vi "二维动态避障简单测试0607(远程版)).vi"() -> ()   [LabVIEW 2018]
doc: "Demonstrates the use of the Network Streams functions to send LED status to the myRIO target."
uses:
  <vilib>/addons/zeromq/socket_type.ctl
  <vilib>/ErrorRing/Error Ring.xnode
  <vilib>/vision/NI_Vision_Development_Module.lvlib
  <vilib>/addons/zeromq/zmq_socket.lvclass
  <vilib>/addons/zeromq/zmq_context.lvclass
  <vilib>/addons/zeromq/zeromq.lvlib
panel:
  in  "start_x手动输入":ext=863.0
  in  "start_y手动输入":ext=497.0
  out "start_point_x 2(opencv判断)":ext
  out "start_point_y 2(opencv判断)":ext
  out "c2":ext
  out "c1":ext
  out "next_relative_desired_point_y":ext
  out "next_relative_desired_point_x":ext
  in  "簇 14":cluster{"c1":ext, "c2":ext}={"c1"=100000.0, "c2"=100000.0}
  out "relative_real_y_color 2":dbl=2.0
  out "relative_real_x_color 2":dbl=2.0
  in  "簇 13":T1={"relative_real_x_color"=100000.0, "relative_real_y_color"=1.0, "t"=1.0}
  out "u(t)_y":ext
  out "u(t)_x":ext
  out "relative_real_y_color":ext
  out "relative_real_x_color":ext
  in  "中心轨迹":bool
  in  "打开彩色点轨迹":bool
  out "relative_real_y_color":ext
  out "relative_real_x_color":ext
  out "彩色轨迹":T2(plugin-control)
  out "end_point_y":ext
  out "end_point_x":ext
  out "end_point_y绝对坐标(opencv拟合)":ext
  out "end_point_x绝对坐标(opencv拟合)":ext
  out "c":ext
  in  "簇 10":T3={"c"=100000.0, "cx"=100000.0, "cy"=100000.0, "start_point_x"=100000.0, "start_point_y"=100000.0}
  out "输出簇":T4
  in  "簇 9":T4={"a"=[], "b"=1.0, "a2"=[], "left1"=1.0, "top1"=1.0, "left2"=1.0, "top2"=1.0, "delta1"=1.0, "delta2"=1.0}
  in  "delta2":dbl=80.0
  out "bottom2":dbl
  out "right2":dbl
  out "top2":dbl
  out "left2":dbl
  in  "delta1":dbl=130.0
  out "bottom1":dbl
  out "right1":dbl
  out "top1":dbl
  out "left1":dbl
  out "delta_pr":dbl
  out "delta_dr":dbl
  in  "k2":dbl=-0.3
  in  "K1":dbl=0.3
  in  "Operation":T5(ring)=enum."Erode"
  out "old_real_relative_point_y":dbl
  out "old_real_relative_point_x":dbl
  out "real_relative_start_point_y":dbl
  out "real_relative_start_point_x":dbl
  out "Bounding Box.Y Top 2":i32
  out "Bounding Box.X Left 2":i32
  out "Ki part":dbl
  out "Kd part":dbl
  out "Kp part":dbl
  out "Ki part":dbl
  out "Kd part":dbl
  out "Kp part":dbl
  in  "Ki":dbl=0.004
  in  "Kd":dbl=5e-05
  in  "Kp":dbl=0.023
  in  "Ki":dbl=0.0035
  in  "Kd":dbl=5e-05
  in  "Kp":dbl=0.023
  out "添加的数组":dbl[](array[numeric])
  out "desired_relative_point_y":dbl=820.0
  out "desired_relative_point_x":dbl=730.0
  out "MLP_pr":dbl=20.0
  out "MLP_dr":dbl=8.0
  out "error_relative_point_y":dbl
  out "error_relative_point_x":dbl
  out "real_relative_end_point_y":dbl
  out "real_relative_end_point_x":dbl
  out "magnet_input_pr":dbl
  out "magnet_input_dr":dbl
  in  "打开仅尖端轨迹":bool
  out "仅尖端轨迹":T2(plugin-control)
  out "Bounding Box.Y Top":i32
  out "Bounding Box.X Left":i32
  out "curve_min_y":dbl
  out "curve_min_x":dbl
  out "curve_max_y":dbl
  out "curve_max_x":dbl
  out "relative_end_point_y":dbl
  out "relative_end_point_x":dbl
  out "delta_y":dbl
  out "delta_x":dbl
  out "pr":dbl=-28.0
  out "tan(v)":dbl
  out "delta_velocity":dbl format="%#_10g"
  out "delta_time":dbl
  out "now time":timestamp[](array[timestamp])
  out "prev time":timestamp[](array[timestamp])
  out "delta_distance":dbl
  out "prev_end_point_y":dbl
  out "prev_end_point_x":dbl
  out "now_end_point_y(曲线拟合)":dbl
  out "now_end_point_x(曲线拟合)":dbl
  out "prev_end_point_y":dbl[](array[numeric])
  out "prev_end_point_x":dbl[](array[numeric])
  out "dr":dbl=120.0
  in  "Ar":sgl=11.0
  out "all parameters":dbl[][](array[numeric])
  out "direction angle":sgl[](array[numeric])
  out "dr":sgl
  out "strength":dbl[](array[numeric])
  out "场强":dbl
  out "end_point_y":T6
  out "end_point_x":dbl[](array[numeric])
  out "start_point_y":dbl[](array[numeric])
  out "start_point_x":dbl[](array[numeric])
  out "T":i32[](array[numeric])
  out "c":dbl[](array[numeric])
  out "b":dbl[](array[numeric])
  out "a\na":dbl[](array[numeric])
  out "c":dbl
  out "b":dbl
  out "a":dbl
  out "Angles (deg)":sgl[](array[numeric]) format="%.2f"
  in  "wr":sgl
  in  "打开轨迹":bool
  out "中心轨迹和尖端轨迹":T2(plugin-control)
  out "end_y绝对坐标(曲线拟合)":dbl
  out "end_x绝对坐标(曲线拟合)":dbl
  out "start_y绝对坐标(曲线拟合)":dbl
  out "start_x绝对坐标(曲线拟合)":dbl
  out "Image Pixels (U8)":u8[][](array[numeric])
  in  "Poly":dbl
  out "中心轨迹":T2(plugin-control)
  in  "保存按钮":bool
  out "Object Center":cluster{"X":sgl, "Y":sgl}
  out "黑白图":T2(plugin-control)
  in  "Number of Erosion":i32=5
  in  "Settings":T7={"Objects"=1, "Threshold"=128, "Reject Border"=FALSE, "Fill Holes"=FALSE, "Min Object Size"=TRUE, "Min Size"=1200, "Max Object Size"=FALSE, "Max Size"=100, "Show Search Area"=TRUE, "Show Center"=TRUE, "Show Bounding Box"=TRUE} {"Objects" items=["Bright Objects", "Dark Objects"]; "Threshold" min=1 max=999999999 step=1; "Max Size" min=1 max=999999999 step=1; "Min Size" min=1 max=999999999 step=1}
  out "Objects":T8(array[cluster]) {"Aspect Ratio" format="%.2f"; "Orientation" format="%.2f"; "Area" format="%.2f"; "Object Center"."Y" format="%.2f"; "Object Center"."X" format="%.2f"}
  in  "Search Rect (entire image)":T9={"Left"=350, "Top"=20, "Right"=1040, "Bottom"=1030, "Rotation"=0.0} {"Rotation" format="%.2f"; "Left" scale=0.0..1024.0; "Right" scale=0.0..1024.0}
  in  "Range":cluster{"Lower value":sgl, "Upper value":sgl}={"Lower value"=177.0, "Upper value"=255.0} {"Upper value" format="%.2f"; "Lower value" format="%.2f"}
  out "原图":T2(plugin-control)
  in  "停止":bool
  out "T":i32
  out "T":i32
  in  "磁场变换":bool=TRUE
  in  "Pause":bool
  out "Array":ext[](array[numeric])
  in  "Parameter Settings":T10(tab)=enum."Rotating Field" caption="Field Types"
  in  "Ag":dbl
  in  "dg":dbl
  in  "pg":dbl
  in  "fg":dbl
  in  "AoOF":dbl
  in  "fo":sgl
  in  "do":sgl
  in  "oo":sgl
  in  "po":sgl
  in  "cc":sgl
  in  "pc":sgl
  in  "wc":sgl
  in  "dc":sgl
  in  "Ac":dbl
  in  "Dis phase step":dbl
  in  "Dis phase frequency (Hz)":dbl
  in  "Dis tumbling frequency (Hz)":dbl
  in  "Dis strength(mT)":dbl
  in  "Swa strength (mT)":dbl
  in  "Swa frequency (Hz)":dbl
  in  "Swa pitch angle (deg)":dbl
  in  "Swa direction angle (deg)":dbl
  in  "Swa ratio":dbl=1.0
  in  "Pitch Angle (rotating around Constant, deg)":dbl
  in  "Ratio (A/C)":sgl
  in  "Direction Angle (deg)":sgl
  in  "Pitch Angle (rotating around Origin, deg)":sgl
  in  "Frequency (Hz)":sgl
  in  "Strength (mT)":dbl
  in  "Ar 2":dbl caption="Ar"
  in  "ratio":sgl
  in  "pr  2":sgl
  in  "dr  2":sgl
  in  "wr  2":sgl
  in  "p_x":sgl
  out "Numeric 5":i32
  in  "Stop":bool
  out "error out":errorcluster
  in  "Target IP Address":string="172.22.11.2"
  # "Overview: Magnetic field calculation, and send parameters to myRIO\nInstructions:\n1. Verify the value of Target IP Address. Set Visa resource name.\n2. Ensure RT Main.vi is already running. \n3. Run this VI. Set parameters of magnetic field."
  # "Strength (mT)"
  # "Frequency (Hz)"
  # "Pitch Angle (deg)"
  # "Direction Angle (deg)"
  # "Strength (mT)"
  # "Pitch Angle (deg)"
  # "Direction Angle (deg)"
  # "Frequency (Hz)"
  # "Strength (mT)"
  # "Oscilation Frequency (Hz)"
  # "Oscilation Angle (deg)"
  # "Pitch Angle (deg)"
  # "Direction Angle (deg)"
  # "Strength (mT)"
  # "Frequency (Hz)"
  # "Pitch Angle (deg)"
  # "Direction Angle (deg)"
  # "Conical Angle (deg)"
  # "Strength (mT)"
  # "Tumbling Frequency (Hz)"
  # "Phase Frequency (Hz)"
  # "Phase Step"
  # "Strength (mT)"
  # "Frequency (Hz)"
  # "Pitch Angle (deg)"
  # "Direction Angle (deg)"
  # "Ratio"
  # "Strength (mT)"
  # "Frequency (Hz)"
  # "Ratio (A/C)"
  # "Direction Angle (deg)"
  # "Pitch Angle (rotating around Origin, deg)"
  # "Pitch Angle (rotating around Constant, deg)"
  # "Strength (mT)"
  # "Frequency (Hz)"
  # "Pitch Angle Y (deg)"
  # "Pitch Angle X (deg)"
  # "Direction Angle (deg)"
  # "ratio (l/s)"
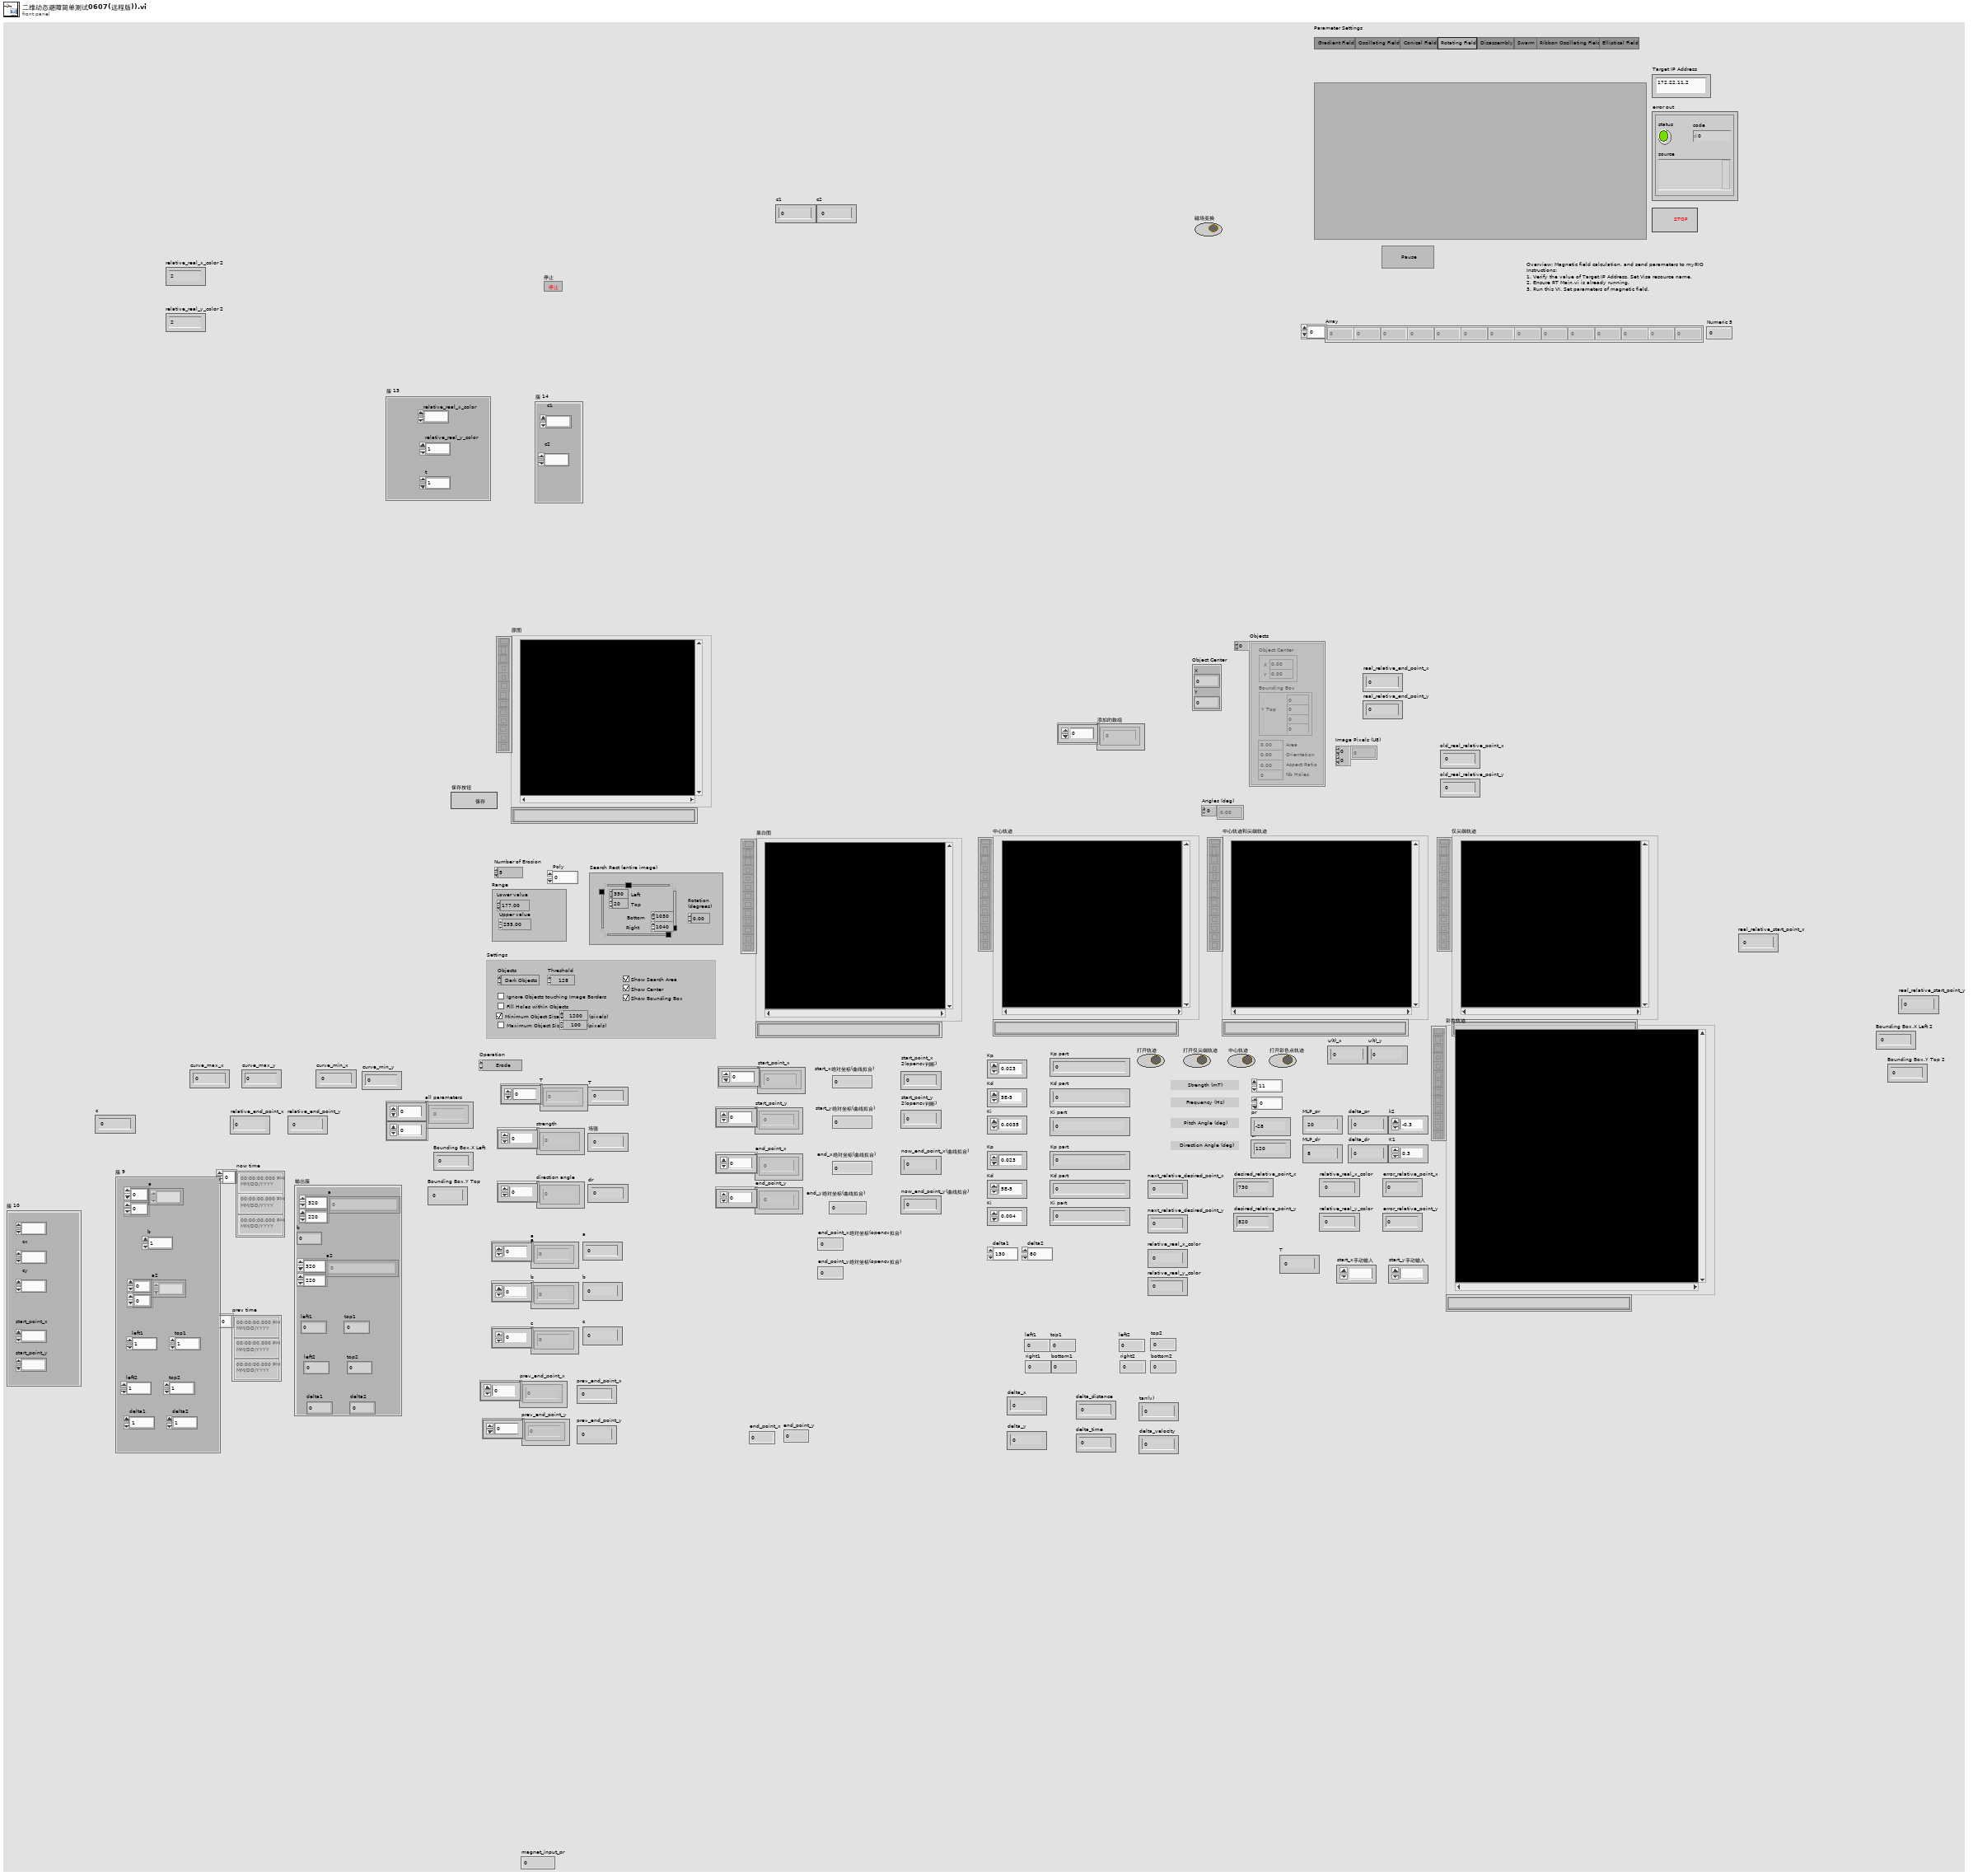
[diagram p1: front panel]
types:
  T1 = cluster{"relative_real_x_color":ext, "relative_real_y_color":dbl, "t":dbl}
  T2 = typedef "IMAQ Image.ctl" = refnum<image>
  T3 = cluster{"c":ext, "cx":ext, "cy":ext, "start_point_x":ext, "start_point_y":ext}
  T4 = cluster{"a":ext[][], "b":dbl, "a2":ext[][], "left1":dbl, "top1":dbl, "left2":dbl, "top2":dbl, "delta1":dbl, "delta2":dbl}
  T5 = enum32{"AutoM", "Close", "Dilate", "Erode", "Gradient", "Gradient in", "Gradient out", "HitMiss", "Open", "PClose", "POpen", "Thick", "Thin"}
  T6 = typedef "控件 3.ctl" = dbl[]
  T7 = cluster{"Objects":u16, "Threshold":i32, "Reject Border":bool, "Fill Holes":bool, "Min Object Size":bool, "Min Size":i32, "Max Object Size":bool, "Max Size":i32, "Show Search Area":bool, "Show Center":bool, "Show Bounding Box":bool}
  T8 = cluster{"Object Center":cluster{"X":sgl, "Y":sgl}, "Bounding Box":cluster{"X Left":i32, "Y Top":i32, "X Right":i32, "Y Bottom":i32}, "Area":sgl, "Orientation":sgl, "Aspect Ratio":sgl, "Nb Holes":i32}[]
  T9 = typedef "IMAQ Rectangle" = cluster{"Left":i32, "Top":i32, "Right":i32, "Bottom":i32, "Rotation":dbl}
  T10 = enum32{"Gradient Field ", "Oscillating Field", "Conical Field", "Rotating Field", "Disassembly", "Swarm", "Ribbon Oscillating Field", "Elliptical Field"}
  T11 = typedef "zeromq.lvlib/socket_type.ctl" = enum8{"ZMQ_PAIR", "ZMQ_PUB", "ZMQ_SUB", "ZMQ_REQ", "ZMQ_REP", "ZMQ_DEALER", "ZMQ_ROUTER", "ZMQ_PULL", "ZMQ_PUSH", "ZMQ_XPUB", "ZMQ_XSUB", "ZMQ_STREAM", "ZMQ_SERVER", "ZMQ_CLIENT", "ZMQ_RADIO", "ZMQ_DISH", "ZMQ_GATHER", "ZMQ_SCATTER", "ZMQ_DGRAM"}
  T12 = typedef "Image Type" = u32
  T13 = cluster{"Object Center":cluster{"X":sgl, "Y":sgl}, "Bounding Box":cluster{"X Left":i32, "Y Top":i32, "X Right":i32, "Y Bottom":i32}, "Area":sgl, "Orientation":sgl, "Aspect Ratio":sgl, "Nb Holes":i32}
  T14 = cluster{"X Left":i32, "Y Top":i32, "X Right":i32, "Y Bottom":i32, "Rotation":dbl}
  T15 = typedef "ROI Descriptor" = cluster{"Global Rectangle":i32[], "Contours":cluster{"ID":enum32{"External", "Internal"}, "Type":u32, "Coordinates":i32[]}[]}
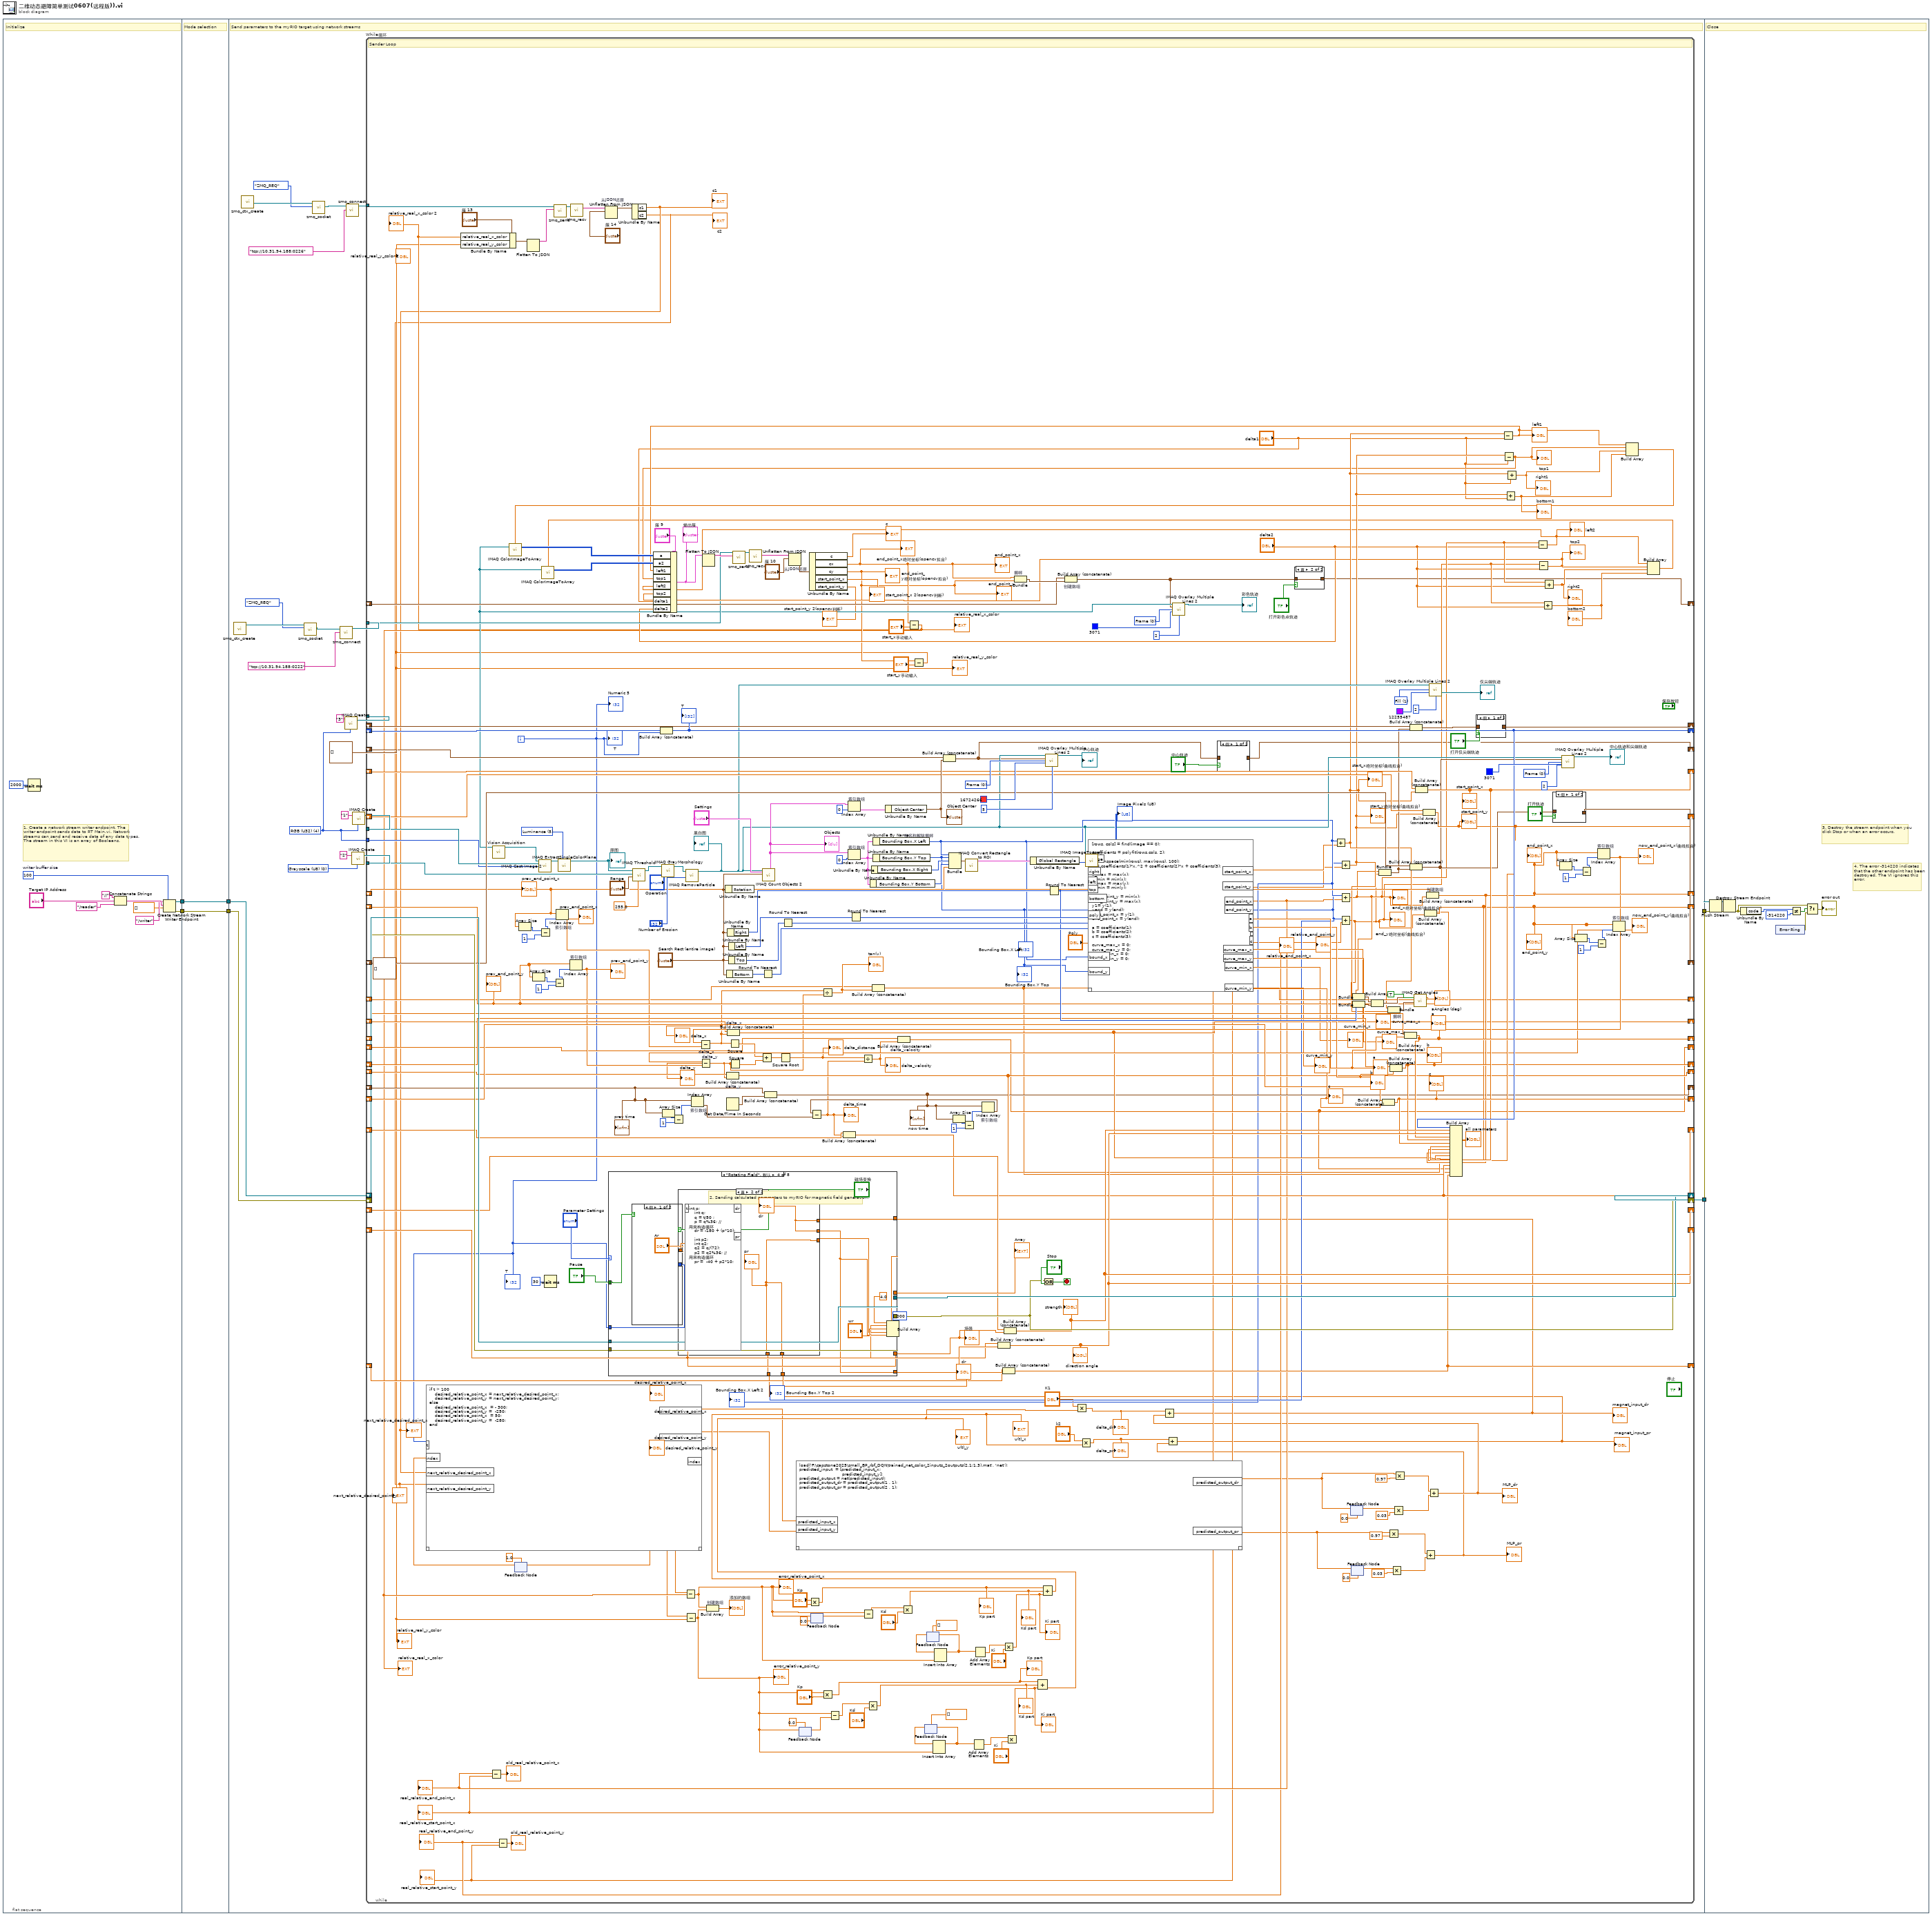
[diagram p0: block diagram]
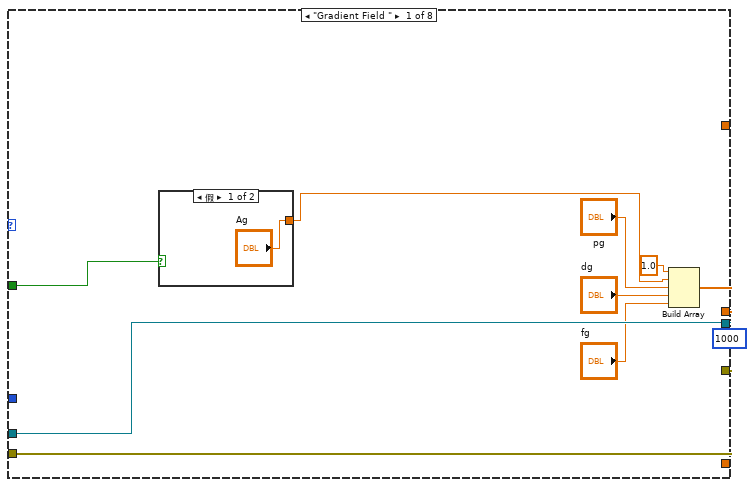
[diagram p6: hidden frame]
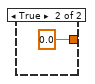
[diagram p7: hidden frame]
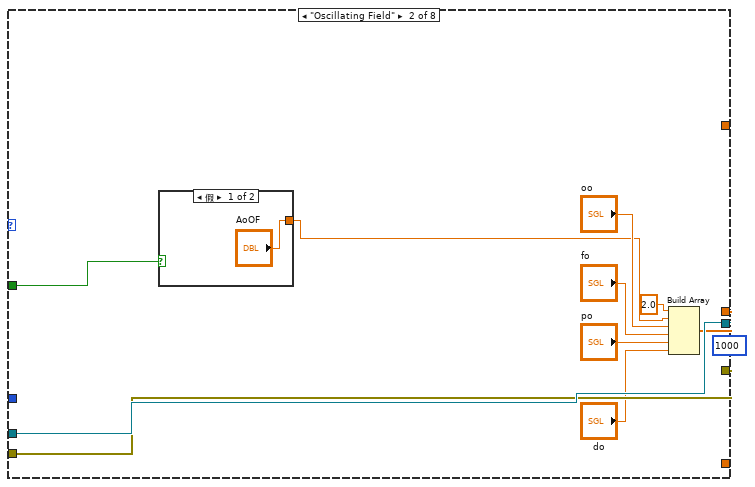
[diagram p8: hidden frame]
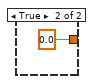
[diagram p9: hidden frame]
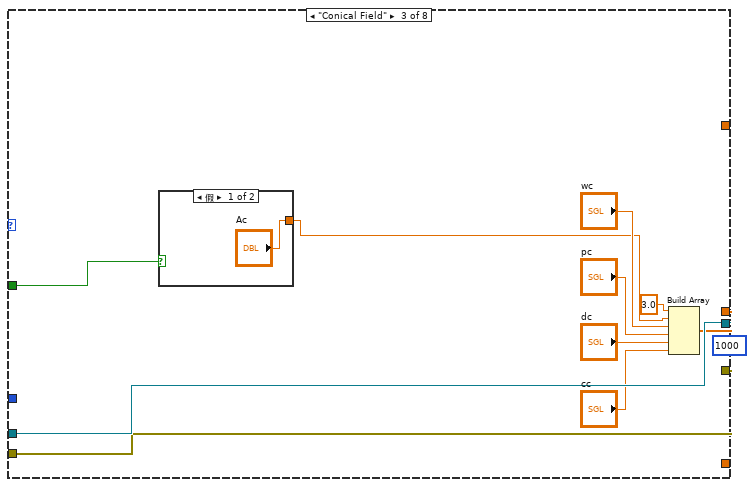
[diagram p10: hidden frame]
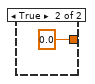
[diagram p11: hidden frame]
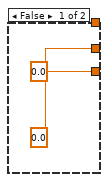
[diagram p12: hidden frame]
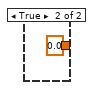
[diagram p13: hidden frame]
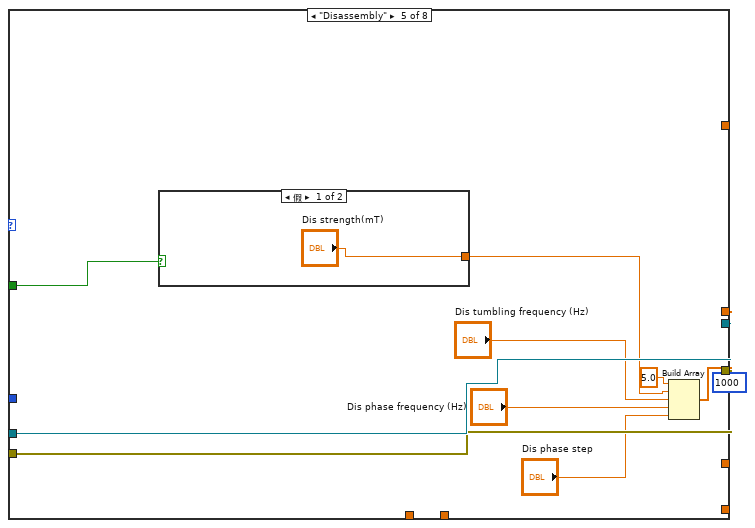
[diagram p14: hidden frame]
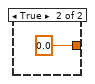
[diagram p15: hidden frame]
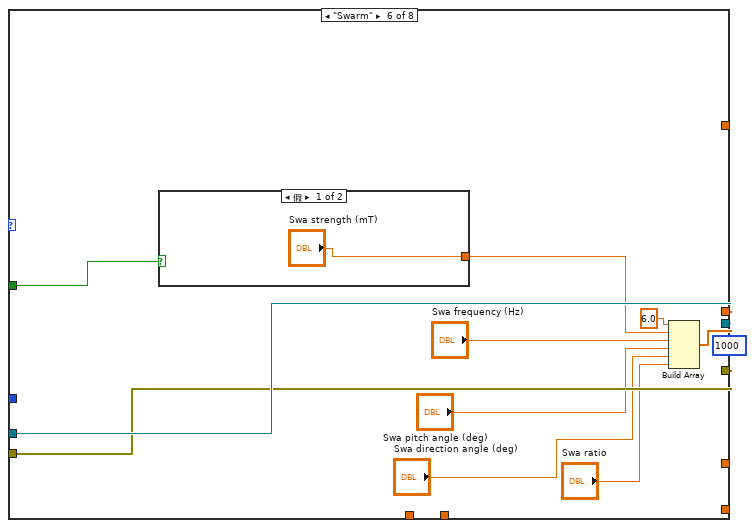
[diagram p16: hidden frame]
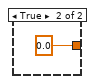
[diagram p17: hidden frame]
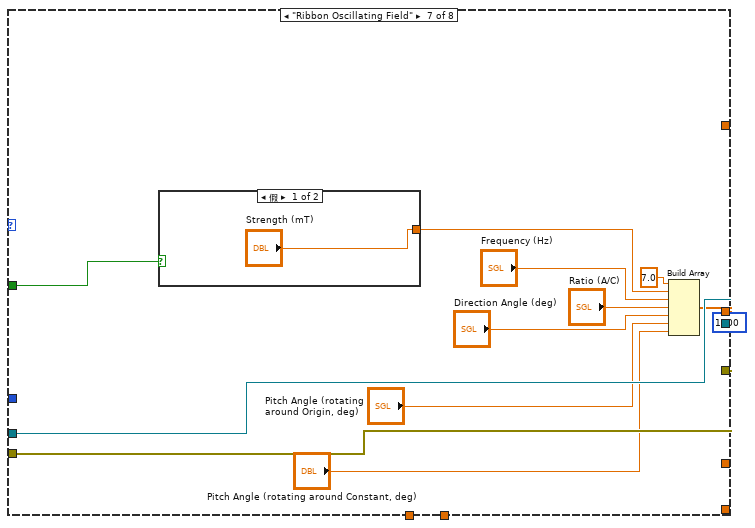
[diagram p18: hidden frame]
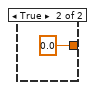
[diagram p19: hidden frame]
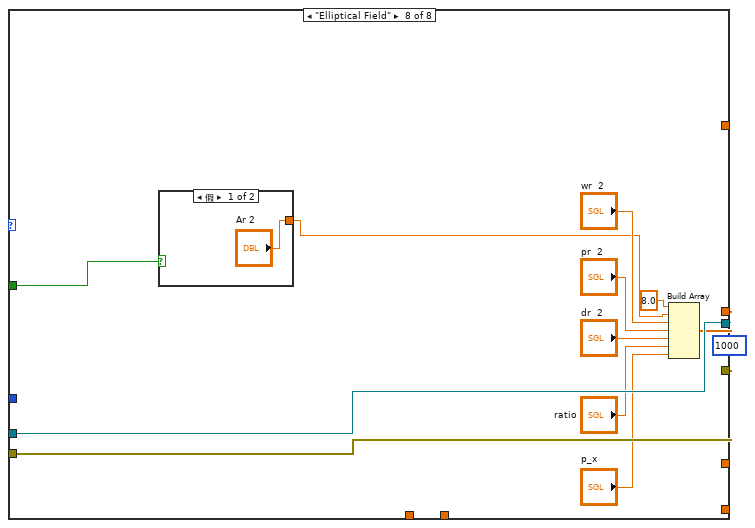
[diagram p20: hidden frame]
diagram:
  n1 = flat-sequence {
    tunnel: [w11] -> w2
    tunnel: [w10] -> w1
    tunnel: [w18] -> w4
    tunnel: [w17] -> w3
    tunnel: w1 -> [w17]
    tunnel: w2 -> [w18]
    tunnel: [w40] -> w6
    tunnel: w4 -> [w42]
    tunnel: [w39] -> w5
    tunnel: w3 -> [w41]
    tunnel: w6 -> [w464]
    tunnel: w5 -> [w461]
    frame #0 {
      w9 = 100  # writer buffer size
      # "1. Create a network stream writer endpoint. The writer endpoint sends data to RT Main.vi. Network streams can send and receive data of any data types. The stream in this VI is an array of Booleans."
      # "Initialize"
      n2 = Wait (ms)(milliseconds to wait=2000) -> ()  [unwired: 1 out]
      n3 = Concatenate Strings("//", "Target IP Address", "/reader") -> (w16:string)
      n4 = Create Network Stream Writer Endpoint(7:w9, 9:dbl[] [], 10:w16, 11:"/writer" ("reader name")) -> (0:w10:errorcluster, 3:w11:refnum<k21>)  [unwired: 3 in]
    }
    frame #1 {
      # "Mode selection"
    }
    frame #2 {
      w36 = T12 0 items=["Grayscale (U8)", "Grayscale (I16)", "Grayscale (SGL)", "Complex (CSG)", "RGB (U32)", "HSL (U32)", "RGB (U64)", "Grayscale (U16)"] ("Image Type")
      w29 = T12 4 items=["Grayscale (U8)", "Grayscale (I16)", "Grayscale (SGL)", "Complex (CSG)", "RGB (U32)", "HSL (U32)", "RGB (U64)", "Grayscale (U16)"] ("Image Type")
      # "Send parameters to the myRIO target using network streams"
      n5 = call <vilib>:"zmq_ctx_create.vi"() -> ("context out"=w27:refnum<class "zmq_context.lvclass">)  [unwired: 4 in, 1 out]
      n6 = call <vilib>:"zmq_ctx_create.vi"() -> ("context out"=w22:refnum<class "zmq_context.lvclass">)  [unwired: 4 in, 1 out]
      n7 = call <vilib>:"zmq_socket.vi"("socket type"=socket_type."ZMQ_REQ", "context in"=w27) -> ("socket out"=w28:refnum<class "zmq_socket.lvclass">)  [unwired: 3 in, 2 out]
      n8 = call <vilib>:"zmq_socket.vi"("socket type"=socket_type."ZMQ_REQ", "context in"=w22) -> ("socket out"=w23:refnum<class "zmq_socket.lvclass">)  [unwired: 3 in, 2 out]
      n9 = call <vilib>:"zmq_connect.vi"("endpoint"="tcp://10.31.94.188:0222", "socket in"=w28) -> ("socket out"=w24:refnum<class "zmq_socket.lvclass">)  [unwired: 2 in, 1 out]
      n10 = call "IMAQ Create"("Image Name"="3", "Image Type"=w29) -> ("New Image"=w32:T2)  [unwired: 3 in, 1 out]
      n11 = call <vilib>:"zmq_connect.vi"("endpoint"="tcp://10.31.94.188:0226", "socket in"=w23) -> ("socket out"=w19:refnum<class "zmq_socket.lvclass">)  [unwired: 2 in, 1 out]
      n12 = call "IMAQ Create"("Image Name"="2", "Image Type"=w36) -> ("New Image"=w34:T2)  [unwired: 3 in, 1 out]
      n13 = call "IMAQ Create"("Image Name"="1", "Image Type"=w29) -> ("New Image"=w35:T2)  [unwired: 3 in, 1 out]
      n14 = while "While循环" {
        shift-right: [w317] -> w39
        shift-left: w41 -> [w319]
        shift-right: [w318] -> w40
        shift-left: w42 -> [w320]
        tunnel: w35 -> [w273]
        tunnel: w34 -> [w272]
        tunnel: w32 -> [_]
        shift-right: [w269] -> _
        shift-left: cluster{"X":dbl, "Y":dbl}[] [] -> [w274]
        shift-right: [w65] -> _
        shift-left: cluster{"X":dbl, "Y":dbl}[] [] -> [w275]
        tunnel: w29 -> [w271]
        shift-right: [w245] -> _
        shift-left: _ -> [w261]
        shift-right: [w240] -> _
        shift-left: _ -> [w259]
        shift-right: [w244] -> _
        shift-left: _ -> [w256]
        shift-right: [w248] -> _
        shift-left: _ -> [w255]
        shift-right: [w243] -> _
        shift-left: _ -> [w254]
        shift-right: [w242] -> _
        shift-left: _ -> [w253]
        shift-right: [w236] -> _
        shift-left: _ -> [w228]
        shift-right: [w232] -> _
        shift-left: _ -> [w224]
        shift-right: [w247] -> _
        shift-left: _ -> [w251]
        shift-right: [w246] -> _
        shift-left: _ -> [w249]
        shift-right: [w213] -> _
        shift-left: _ -> [w215]
        shift-right: [w212] -> _
        shift-left: _ -> [w214]
        shift-right: [w202] -> _
        shift-left: _ -> [w207]
        shift-right: [w199] -> _
        shift-left: _ -> [w200]
        shift-right: [w195] -> _
        shift-left: _ -> [w196]
        shift-right: [w190] -> _
        shift-left: _ -> [w191]
        shift-right: [w182] -> _
        shift-left: _ -> [w183]
        shift-right: [w176] -> _
        shift-left: _ -> [w177]
        shift-right: [w69] -> _
        shift-left: _ -> [w86]
        tunnel: w24 -> [w84]
        tunnel: w19 -> [w54]
        i -> [w53]
        stop <- w313 stop-if-true
        w94 = u32 0 items=["Frame", "Fill"] ("Drawing Mode (Frame)")
        w178 = u32 1 items=["Frame", "Fill"] ("Drawing Mode (Frame)")
        w185 = u32 0 items=["Frame", "Fill"] ("Drawing Mode (Frame)")
        w300 = u32 0 items=["Frame", "Fill"] ("Drawing Mode (Frame)")
        w310 = 5 items=["Red", "Green", "Blue", "Hue", "Saturation", "Luminance", "Value", "Intensity"] ("Color Plane")
        # "2. Sending calculated parameters to myRIO for magnetic field generation."
        # "Sender Loop"
        n15 = call "Vision Acquisition"() -> ("Image Out"=w83:T2)  [unwired: 23 in, 4 out]
        n16 = feedback #1(1.0) -> (w80:dbl)
        n17 = Array Size(array=w228) -> (size(s)=w230:i32)
        n18 = Array Size(array=w224) -> (size(s)=w226:i32)
        n19 = call "IMAQ Cast Image 2"("Image Src"=w83, "Image Dst"=w273, "Image Type"=w271) -> ("Image Dst Out"=w311:T2)  [unwired: 11 in, 1 out]
        n20 = Subtract(x=w230, y=1) -> (x-y=w229:i32)
        n21 = Wait (ms)(milliseconds to wait=u32 30 ("等待时间（毫秒）")) -> ()  [unwired: 1 out]
        n22 = Subtract(x=w226, y=1) -> (x-y=w225:i32)
        n23 = Index Array "索引数组"(array=w228, index=w229) -> (element=w222:dbl)
        "prev_end_point_x" <- w222
        n24 = call "IMAQ ExtractSingleColorPlane"("Color Plane"=w310, "Image Src"=w311) -> ("Image Dst Out"=w309:T2)  [unwired: 8 in, 1 out]
        "原图" <- w309
        n25 = Index Array "索引数组"(array=w224, index=w225) -> (element=w221:dbl)
        "prev_end_point_y" <- w221
        n26 = call "IMAQ Threshold"("Replace Value"=sgl 255.0, "Range"="Range", "Image Dst"=w272, "Image Src"=w309) -> ("Image Dst Out"=w135:T2)  [unwired: 6 in, 1 out]
        n27 = Build Array (concatenate)(w255, w53) -> (w248:i32[])
        "T" <- w248
        n28 = call "IMAQ GrayMorphology"("Operation"="Operation", "Image Src"=w135) -> ("Image Dst Out"=w134:T2)  [unwired: 8 in, 1 out]
        n29 = Array Size(array=w207) -> (size(s)=w210:i32)
        n30 = Subtract(x=w210, y=1) -> (x-y=w209:i32)
        n31 = call "IMAQ RemoveParticle"("Number of Erosion"="Number of Erosion", "Image Src"=w134) -> ("Image Dst Out"=w174:T2)  [unwired: 8 in, 1 out]
        "黑白图" <- w174
        n32 = Index Array "索引数组"(array=w207, index=w209) -> (element=w206:timestamp)
        n33 = Unbundle By Name("Search Rect (entire image)") -> ("Rotation"=w296:dbl)
        n34 = Unbundle By Name("Search Rect (entire image)") -> ("Bottom"=w280:i32)
        n35 = Get Date/Time In Seconds() -> (seconds since 1Jan1904=w211:timestamp)
        n36 = Unbundle By Name("Search Rect (entire image)") -> ("Right"=w284:i32)
        n37 = Unbundle By Name("Search Rect (entire image)") -> ("Left"=w283:i32)
        n38 = Unbundle By Name("Search Rect (entire image)") -> ("Top"=w282:i32)
        n39 = Round To Nearest(number=w280) -> (nearest integer value=w279:i32)
        n40 = call "IMAQ Count Objects 2"("Settings"="Settings", "Search Rect (entire image)"="Search Rect (entire image)", "Image"=w174) -> ("Objects"=w298:T8)  [unwired: 4 in, 4 out]
        "Objects" <- w298
        n41 = Build Array (concatenate)(w207, w211) -> (w202:timestamp[])
        "now time" <- w202
        n42 = Round To Nearest(number=w282) -> (nearest integer value=w281:i32)
        n43 = feedback #2(0.0) -> (w153:ext)
        n44 = feedback #3(0.0) -> (w167:ext)
        n45 = Index Array "索引数组"(array=w298, index=0 ("索引")) -> (element=w303:T13)
        n46 = Index Array "索引数组"(array=w298, index=0 ("索引")) -> (element=w294:T13)
        n47 = Round To Nearest(number=w283) -> (nearest integer value=w277:i32)
        n48 = Unbundle By Name(w294) -> ("Bounding Box.Y Bottom"=w288:i32)
        n49 = Unbundle By Name(w294) -> ("Bounding Box.X Right"=w289:i32)
        n50 = Unbundle By Name "按名称解除捆绑"(w294) -> ("Bounding Box.X Left"=w141:i32)
        "Bounding Box.X Left" <- w141
        "Bounding Box.X Left 2" <- w141
        n51 = Unbundle By Name(w294) -> ("Bounding Box.Y Top"=w140:i32)
        "Bounding Box.Y Top" <- w140
        "Bounding Box.Y Top 2" <- w140
        n52 = Unbundle By Name(w303) -> ("Object Center"=w302:cluster{"X":sgl, "Y":sgl})
        "Object Center" <- w302
        n53 = feedback #4(dbl[] []) -> (w148:dbl[])
        n54 = feedback #5(dbl[] []) -> (w162:dbl[])
        n55 = Build Array (concatenate)(w275, w302) -> (w66:cluster{"X":dbl, "Y":dbl}[])
        n56 = Bundle("X Left"=w141, "Y Top"=w140, "X Right"=w289, "Y Bottom"=w288, "Rotation"=w296) -> (w295:T14)  [unwired: 1 in]
        n57 = Array Size(array=w202) -> (size(s)=w205:i32)
        n58 = Subtract(x=w205, y=1) -> (x-y=w204:i32)
        n59 = call "IMAQ Convert Rectangle to ROI"("Rectangle"=w295) -> ("ROI Descriptor"=w293:T15)  [unwired: 8 in, 1 out]
        n60 = Index Array "索引数组"(array=w202, index=w204) -> (element=w201:timestamp)
        n61 = Subtract(x=w201, y=w206) -> (x-y=w198:dbl)
        "delta_time" <- w198
        n62 = Build Array (concatenate)(w200, w198) -> (w199:dbl[])
        n63 = Unbundle By Name(w293) -> ("Global Rectangle"=w278:i32[])
        n64 = call "IMAQ Overlay Multiple Lines 2"("Image"=w174, "Line End Points"=w66, "Drawing Mode (Frame)"=w300, "Color"=u32 16724266, "Width"=u32 5) -> ("Image Out"=→"中心轨迹":T2)  [unwired: 9 in, 1 out]
        n65 = Round To Nearest(number=w284) -> (nearest integer value=w262:i32)
        n66 = call "IMAQ ImageToArray"("Optional Rectangle"=w278, "Image"=w174) -> ("Image Pixels (U8)"=w290:u8[][])  [unwired: 2 in, 4 out]
        "Image Pixels (U8)" <- w290
        n67 = script code="[rows, cols] = find(image == 0); \n\ncoefficients = polyfit(rows,cols, 2);\n\nx = linspace(min(rows), max(rows), 100); \ny = coefficients(1)*x.^2 + coefficients(2)*x + coefficients(3);\n\nx_max = max(x);\nx_min = min(x);\ny_max = max(y);\ny_min = min(y);\n\nstart_point_y = min(x);\nend_point_y = max(x);\ny1= y(1);\nyend = y(end);\nstart_point_x = y(1);\nend_point_x = y(end);\n\na = coefficients(1);\nb = coefficients(2);\nc = coefficients(3);\n\ncurve_max_x = 0;\ncurve_max_y = 0;\ncurve_min_x = 0;\ncurve_min_y = 0;"("image"=w290, "poly"="Poly", "right"=w262, "left"=w277, "top"=w281, "bottom"=w279, "bound_x"=w141, "bound_y"=w140) -> ("start_point_x"=w138:dbl, "start_point_y"=w136:dbl, "end_point_x"=w139:dbl, "end_point_y"=w137:dbl, "a"=w260:dbl, "b"=w258:dbl, "c"=w257:dbl, "curve_max_x"=→"curve_max_x":dbl, "curve_max_y"=→"curve_max_y":dbl, "curve_min_x"=→"curve_min_x":dbl, "curve_min_y"=→"curve_min_y":dbl)  [unwired: 1 in, 1 out]
        "a" <- w260
        "b" <- w258
        "c" <- w257
        "relative_end_point_x" <- w139
        "relative_end_point_y" <- w137
        "real_relative_end_point_x" <- w139
        "real_relative_end_point_y" <- w137
        "real_relative_start_point_x" <- w138
        "real_relative_start_point_y" <- w136
        n68 = Subtract(x=w139, y=w138) -> (x-y=→"old_real_relative_point_x":dbl)
        n69 = Subtract(x=w137, y=w136) -> (x-y=→"old_real_relative_point_y":dbl)
        n70 = case shown="假" "中心轨迹" {
          tunnel: w66 -> [_ w322]
          tunnel: [_ w322] -> w65
          frame False {
          }
          frame True {
          }
        }
        n71 = Add(x=w141, y=w138) -> (x+y=w108:dbl)
        "start_x绝对坐标(曲线拟合)" <- w108
        n72 = Add(x=w140, y=w136) -> (x+y=w107:dbl)
        "start_y绝对坐标(曲线拟合)" <- w107
        n73 = Add(x=w141, y=w139) -> (x+y=w106:dbl)
        "end_x绝对坐标(曲线拟合)" <- w106
        n74 = Add(x=w140, y=w137) -> (x+y=w105:dbl)
        "end_y绝对坐标(曲线拟合)" <- w105
        n75 = feedback #6(0.0) -> (w130:dbl)
        n76 = feedback #7(0.0) -> (w122:dbl)
        n77 = Bundle(w106, w105) -> (w266:cluster{dbl, dbl})  [unwired: 1 in]
        n78 = Bundle(w262, w107) -> (w265:cluster{i32, dbl})  [unwired: 1 in]
        n79 = Build Array(w266, w265) -> (w264:cluster{dbl, dbl}[])
        n80 = Bundle(w106, w105) -> (w172:cluster{dbl, dbl})  [unwired: 1 in]
        n81 = Build Array (concatenate)(w256, w257) -> (w244:dbl[])
        "c" <- w244
        n82 = Bundle "捆绑"(w108, w107) -> (w267:cluster{dbl, dbl})  [unwired: 1 in]
        n83 = Build Array (concatenate)(w259, w258) -> (w240:dbl[])
        "b" <- w240
        n84 = Multiply(x=w122, y=0.03) -> (x*y=w119:dbl)
        n85 = Multiply(x=w130, y=0.03) -> (x*y=w126:dbl)
        n86 = Build Array (concatenate)(w261, w260) -> (w245:dbl[])
        "a\na" <- w245
        n87 = Build Array (concatenate)(w274, w172) -> (w173:cluster{"X":dbl, "Y":dbl}[])
        n88 = Build Array (concatenate)(w177, w172) -> (w171:cluster{dbl, dbl}[])
        n89 = call "IMAQ Get Angles"("Vertex"=w267, "Points"=w264, "Use Vertex (No)"=TRUE) -> ("Angles (deg)"=→"Angles (deg)":sgl[])  [unwired: 2 in, 2 out]
        n90 = Build Array (concatenate)(w254, w108) -> (w243:dbl[])
        "start_point_x" <- w243
        n91 = Build Array (concatenate)(w253, w107) -> (w242:dbl[])
        "start_point_y" <- w242
        n92 = Build Array (concatenate)(w224, w105) -> (w232:dbl[])
        "end_point_y" <- w232
        n93 = Build Array (concatenate) "创建数组"(w228, w106) -> (w236:dbl[])
        "end_point_x" <- w236
        n94 = call "IMAQ Overlay Multiple Lines 2"("Image"=w174, "Drawing Mode (Frame)"=w178, "Color"=u32 12255487, "Width"=u32 2) -> ("Image Out"=→"仅尖端轨迹":T2)  [unwired: 10 in, 1 out]
        n95 = case shown="假" "打开仅尖端轨迹" {
          tunnel: [_ w324] -> w176
          tunnel: w171 -> [_ w324]
          frame False {
          }
          frame True {
          }
        }
        n96 = Subtract(x=w108, y="delta1") -> (x-y=w89:dbl)
        "left1" <- w89
        n97 = Subtract(x=w107, y="delta1") -> (x-y=w88:dbl)
        "top1" <- w88
        n98 = Add(x=w107, y="delta1") -> (x+y=w109:dbl)
        "bottom1" <- w109
        n99 = Add(x=w108, y="delta1") -> (x+y=w110:dbl)
        "right1" <- w110
        n100 = Subtract(x=w106, y="delta2") -> (x-y=w87:dbl)
        "left2" <- w87
        n101 = Subtract(x=w105, y="delta2") -> (x-y=w85:dbl)
        "top2" <- w85
        n102 = Add(x=w105, y="delta2") -> (x+y=w111:dbl)
        "bottom2" <- w111
        n103 = Add(x=w106, y="delta2") -> (x+y=w112:dbl)
        "right2" <- w112
        n104 = case shown="假" "打开轨迹" {
          tunnel: [_ w325] -> w269
          tunnel: w173 -> [_ w325]
          frame False {
          }
          frame True {
          }
        }
        n105 = Array Size(array=w236) -> (size(s)=w238:i32)
        n106 = call "IMAQ Overlay Multiple Lines 2"("Image"=w174, "Line End Points"=w173, "Drawing Mode (Frame)"=w185, "Color"=u32 3071, "Width"=u32 2) -> ("Image Out"=→"中心轨迹和尖端轨迹":T2)  [unwired: 9 in, 1 out]
        n107 = Array Size(array=w232) -> (size(s)=w234:i32)
        n108 = Subtract(x=w238, y=1) -> (x-y=w237:i32)
        n109 = Subtract(x=w234, y=1) -> (x-y=w233:i32)
        n110 = Index Array "索引数组"(array=w236, index=w237) -> (element=w223:dbl)
        "now_end_point_x(曲线拟合)" <- w223
        n111 = Subtract "delta_x"(x=w223, y=w222) -> (x-y=w194:dbl)
        "delta_x" <- w194
        n112 = Build Array (concatenate) "delta_x"(w215, w194) -> (w213:dbl[])
        n113 = Square(x=w194) -> (x^2=w219:dbl)
        n114 = Index Array "索引数组"(array=w232, index=w233) -> (element=w220:dbl)
        "now_end_point_y(曲线拟合)" <- w220
        n115 = Subtract "delta_y"(x=w220, y=w221) -> (x-y=w193:dbl)
        "delta_y" <- w193
        n116 = Build Array (concatenate) "delta_y"(w214, w193) -> (w212:dbl[])
        n117 = Square(x=w193) -> (x^2=w218:dbl)
        n118 = Add(x=w219, y=w218) -> (x+y=w217:dbl)
        n119 = Square Root(x=w217) -> (sqrt(x)=w216:dbl)
        "delta_distance" <- w216
        n120 = Divide(x=w194, y=w193) -> (x/y=w192:dbl)
        "tan(v)" <- w192
        n121 = Divide(x=w216, y=w198) -> (x/y=w197:dbl)
        "delta_velocity" <- w197
        n122 = Build Array (concatenate)(w191, w192) -> (w190:dbl[])
        n123 = Build Array (concatenate) "delta_velocity"(w196, w197) -> (w195:dbl[])
        n124 = Build Array(w89, w88, w110, w109) -> (w104:dbl[])
        n125 = call "IMAQ ColorImageToArray"("Optional Rectangle"=w104, "Image"=w83) -> ("Image Pixels (U32)"=w91:u32[][])  [unwired: 2 in, 2 out]
        n126 = Build Array(w87, w85, w112, w111) -> (w62:dbl[])
        n127 = call "IMAQ ColorImageToArray"("Optional Rectangle"=w62, "Image"=w83) -> ("Image Pixels (U32)"=w90:u32[][])  [unwired: 2 in, 2 out]
        n128 = Bundle By Name(cluster="簇 9", "a"=w91, "a2"=w90, "left1"=w89, "top1"=w88, "left2"=w87, "top2"=w85, "delta1"="delta1", "delta2"="delta2") -> (w97:T4)
        "输出簇" <- w97
        n129 = Flatten To JSON(anything=w97) -> (JSON string=w96:string)  [unwired: 2 in, 1 out]
        n130 = call <vilib>:"zmq_send.vi"("data"=w96, "socket in"=w84) -> ("socket out"=w101:refnum<class "zmq_socket.lvclass">)  [unwired: 5 in, 1 out]
        n131 = call <vilib>:"zmq_recv.vi"("socket in"=w101) -> ("data"=w102:string)  [unwired: 4 in, 4 out]
        n132 = Unflatten From JSON "从JSON还原"(JSON string=w102, type and defaults="簇 10") -> (value=w99:T3)  [unwired: 5 in, 1 out]
        n133 = Unbundle By Name(w99) -> ("c"=→"c":ext, "cx"=w74:ext, "cy"=w72:ext, "start_point_x"=→"start_point_x 2(opencv判断)":ext, "start_point_y"=→"start_point_y 2(opencv判断)":ext)
        "end_point_x绝对坐标(opencv拟合)" <- w74
        "end_point_y绝对坐标(opencv拟合)" <- w72
        "end_point_x" <- w74
        "end_point_y" <- w72
        n134 = Subtract(x=w74, y="start_x手动输入") -> (x-y=w52:ext)
        "relative_real_x_color" <- w52
        "relative_real_x_color" <- w52
        "relative_real_x_color 2" <- w52
        n135 = Subtract(x=w72, y="start_y手动输入") -> (x-y=w51:ext)
        "relative_real_y_color" <- w51
        "relative_real_y_color" <- w51
        "relative_real_y_color 2" <- w51
        n136 = Bundle By Name(cluster="簇 13", "relative_real_x_color"=w52, "relative_real_y_color"=w51) -> (w60:T1)
        n137 = Flatten To JSON(anything=w60) -> (JSON string=w55:string)  [unwired: 2 in, 1 out]
        n138 = call <vilib>:"zmq_send.vi"("data"=w55, "socket in"=w54) -> ("socket out"=w58:refnum<class "zmq_socket.lvclass">)  [unwired: 5 in, 1 out]
        n139 = call <vilib>:"zmq_recv.vi"("socket in"=w58) -> ("data"=w59:string)  [unwired: 4 in, 4 out]
        n140 = Unflatten From JSON "从JSON还原"(JSON string=w59, type and defaults="簇 14") -> (value=w56:cluster{"c1":ext, "c2":ext})  [unwired: 5 in, 1 out]
        n141 = Unbundle By Name(w56) -> ("c1"=w50:ext, "c2"=w49:ext)
        "next_relative_desired_point_x" <- w50
        "next_relative_desired_point_y" <- w49
        "c1" <- w50
        "c2" <- w49
        n142 = script code="if t > 100\n    desired_relative_point_x = next_relative_desired_point_x;\n    desired_relative_point_y = next_relative_desired_point_y;\nelse\n    desired_relative_point_x  = - 300;\n    desired_relative_point_y =  -250;\n    desired_relative_point_x  = 50;\n    desired_relative_point_y =  -280;\nend"("t"=w53, "index"=w80, "next_relative_desired_point_x"=w50, "next_relative_desired_point_y"=w49) -> ("desired_relative_point_x"=w48:dbl, "desired_relative_point_y"=w47:dbl, "index"=w81:dbl)  [unwired: 1 in, 1 out]
        "desired_relative_point_x" <- w48
        "desired_relative_point_y" <- w47
        n143 = feedback-in #1(w81) -> ()
        n144 = Subtract(x=w48, y=w52) -> (x-y=w161:ext)
        "error_relative_point_x" <- w161
        n145 = Subtract(x=w47, y=w51) -> (x-y=w146:ext)
        "error_relative_point_y" <- w146
        n146 = Build Array "创建数组"(w161, w146) -> (→"添加的数组":ext[])
        n147 = script code="load('F:\\capstone2025\\small_BP_rbf_DQN\\trained_net_color_2inputs_2outputs(2.1;1.3).mat', 'net');\npredicted_input  = [predicted_input_x; \n                               predicted_input_y];\npredicted_output = net(predicted_input);\npredicted_output_dr = predicted_output(1 , 1);\npredicted_output_pr = predicted_output(2 , 1);"("predicted_input_y"=w47, "predicted_input_x"=w48) -> ("predicted_output_dr"=w131:dbl, "predicted_output_pr"=w124:dbl)  [unwired: 1 in, 1 out]
        n148 = feedback-in #2(w146) -> ()
        n149 = Multiply(x=w161, y="Kp") -> (x*y=w168:ext)
        "Kp part" <- w168
        n150 = feedback-in #3(w161) -> ()
        n151 = Multiply(x=w146, y="Kp") -> (x*y=w154:ext)
        "Kp part" <- w154
        n152 = Subtract(x=w146, y=w153) -> (x-y=w151:ext)
        n153 = Subtract(x=w161, y=w167) -> (x-y=w165:ext)
        n154 = Multiply(x=w151, y="Kd") -> (x*y=w149:ext)
        "Kd part" <- w149
        n155 = Multiply(x=w165, y="Kd") -> (x*y=w163:ext)
        "Kd part" <- w163
        n156 = Insert Into Array(array=w148, new element=w146) -> (w147:dbl[])  [unwired: 1 in]
        n157 = feedback-in #4(w147) -> ()
        n158 = Insert Into Array(array=w162, new element=w161) -> (w160:dbl[])  [unwired: 1 in]
        n159 = feedback-in #5(w160) -> ()
        n160 = Add Array Elements(numeric array=w147) -> (sum=w144:dbl)
        n161 = Add Array Elements(numeric array=w160) -> (sum=w158:dbl)
        n162 = Multiply(x=w158, y="Ki") -> (x*y=w156:dbl)
        "Ki part" <- w156
        n163 = Multiply(x=w144, y="Ki") -> (x*y=w142:dbl)
        "Ki part" <- w142
        n164 = Bundle "捆绑"("cx"=w74, "cy"=w72) -> (w95:cluster{"cx":ext, "cy":ext})  [unwired: 1 in]
        n165 = Compound Arithmetic op=ADD(w154, w149, w142) -> (w63:ext)
        "u(t)_y" <- w63
        n166 = Compound Arithmetic op=ADD(w168, w163, w156) -> (w64:ext)
        "u(t)_x" <- w64
        n167 = Build Array (concatenate) "创建数组"(w86, w95) -> (w70:cluster{"cx":ext, "cy":ext}[])
        n168 = Multiply(x="K1", y=w63) -> (x*y=w46:ext)
        "delta_dr" <- w46
        n169 = Multiply(x="k2", y=w64) -> (x*y=w45:ext)
        "delta_pr" <- w45
        n170 = call "IMAQ Overlay Multiple Lines 2"("Image"=w83, "Line End Points"=w70, "Drawing Mode (Frame)"=w94, "Color"=u32 3071, "Width"=u32 2) -> ("Image Out"=→"彩色轨迹":T2)  [unwired: 9 in, 1 out]
        n171 = case shown="真" "打开彩色点轨迹" {
          tunnel: [_ w323] -> w69
          tunnel: w70 -> [_ w323]
          frame False {
          }
          frame True {
          }
        }
        n172 = feedback-in #6(w131) -> ()
        n173 = feedback-in #7(w124) -> ()
        n174 = Multiply(x=w124, y=0.97) -> (x*y=w120:dbl)
        n175 = Multiply(x=w131, y=0.97) -> (x*y=w127:dbl)
        n176 = Add(x=w120, y=w119) -> (x+y=w117:dbl)
        "MLP_pr" <- w117
        n177 = Add(x=w45, y=w117) -> (x+y=w115:ext)
        "magnet_input_pr" <- w115
        n178 = Add(x=w127, y=w126) -> (x+y=w118:dbl)
        "MLP_dr" <- w118
        n179 = Add(x=w46, y=w118) -> (x+y=w116:ext)
        "magnet_input_dr" <- w116
        n180 = case shown="\"Rotating Field\", 默认" "Parameter Settings" {
          tunnel: w320 -> [w336 w351 w366 w385 w404 w418 w436 w451]
          tunnel: w319 -> [w333 w350 w365 w384 w402 w417 w434 w450]
          tunnel: [w335 w349 w363 w383 w403 w416 w435 w449] -> w318
          tunnel: [w334 w348 w364 w382 w401 w415 w433 w448] -> w317
          tunnel: [w329 w342 w357 w378 w395 w410 w431 w443] -> w316
          tunnel: "Pause" -> [w327 w340 w355 w377 w394 w409 w426 w441]
          tunnel: [_ _ _ w374 _ _ _ _] -> w252
          tunnel: [_ _ _ w375 _ _ _ _] -> w250
          tunnel: w53 -> [_ _ _ w373 _ _ _ _]
          tunnel: [_ _ _ w372 _ _ _ _] -> w184
          tunnel: w116 -> [_ _ _ w371 _ _ _ _]
          tunnel: w115 -> [_ _ _ w370 _ _ _ _]
          frame "Gradient Field " {
            n181 = case shown="假" w327 {
              tunnel: ["Ag" 0.0] -> w328
              frame False {
              }
              frame True {
              }
            }
            n182 = Build Array(1.0, w328, "pg", "dg", "fg") -> (w329:dbl[])
            n183 = shared-variable-write(w336, w333, w329, 1000 ("timeout ms (-1)")) -> (w335:refnum<k21>, w334:errorcluster)  [unwired: 1 out]
          }
          frame "Oscillating Field" {
            n184 = case shown="假" w340 {
              tunnel: ["AoOF" 0.0] -> w341
              frame False {
              }
              frame True {
              }
            }
            n185 = Build Array(2.0, w341, "oo", "fo", "po", "do") -> (w342:dbl[])
            n186 = shared-variable-write(w351, w350, w342, 1000 ("timeout ms (-1)")) -> (w349:refnum<k21>, w348:errorcluster)  [unwired: 1 out]
          }
          frame "Conical Field" {
            # "FG"
            n187 = case shown="假" w355 {
              tunnel: ["Ac" 0.0] -> w356
              frame False {
              }
              frame True {
              }
            }
            n188 = Build Array(3.0, w356, "wc", "pc", "dc", "cc") -> (w357:dbl[])
            n189 = shared-variable-write(w366, w365, w357, 1000 ("timeout ms (-1)")) -> (w363:refnum<k21>, w364:errorcluster)  [unwired: 1 out]
          }
          frame "Rotating Field", Default {
            n190 = case shown="假" w377 {
              tunnel: ["Ar" 0.0] -> w374
              frame False {
              }
              frame True {
              }
            }
            n191 = case shown="真" "磁场变换" {
              tunnel: [sgl 0.0 ("pr") w389] -> w380
              tunnel: [sgl 0.0 ("dr") w390] -> w375
              tunnel: w373 -> [_ w391]
              tunnel: [_ w389] -> w372
              tunnel: w371 -> [_ w390]
              tunnel: w370 -> [_ w389]
              frame False {
              }
              frame True {
                n192 = formula code="int p;\n    int q;\n    q = t/50 ;  \n    p = q%36; //用来构造循环\n    dr = -180 + (p*10);\n\n    int p2;\n    int q2;\n    q2 = q/(72);\n    p2 = q2%36; //用来构造循环\n    pr =  -40 + p2*10;"("t"=w391) -> ()  [unwired: 2 out]
                "dr" <- w390
                "pr" <- w389
              }
            }
            n193 = Build Array(4.0, w374, "wr", w380, w375) -> (w378:ext[])
            n194 = shared-variable-write "向流中写入单个元素"(w385, w384, w378, 1000 ("timeout ms (-1)")) -> (w383:refnum<k21>, w382:errorcluster)  [unwired: 1 out]
          }
          frame "Disassembly" {
            n195 = case shown="假" w394 {
              tunnel: ["Dis strength(mT)" 0.0] -> w399
              frame False {
              }
              frame True {
              }
            }
            n196 = Build Array(5.0, w399, "Dis tumbling frequency (Hz)", "Dis phase frequency (Hz)", "Dis phase step") -> (w395:dbl[])
            n197 = shared-variable-write(w404, w402, w395, 1000 ("timeout ms (-1)")) -> (w403:refnum<k21>, w401:errorcluster)  [unwired: 1 out]
          }
          frame "Swarm" {
            n198 = case shown="假" w409 {
              tunnel: ["Swa strength (mT)" 0.0] -> w408
              frame False {
              }
              frame True {
              }
            }
            n199 = Build Array(6.0, w408, "Swa frequency (Hz)", "Swa pitch angle (deg)", "Swa direction angle (deg)", "Swa ratio") -> (w410:dbl[])
            n200 = shared-variable-write(w418, w417, w410, 1000 ("timeout ms (-1)")) -> (w416:refnum<k21>, w415:errorcluster)  [unwired: 1 out]
          }
          frame "Ribbon Oscillating Field" {
            n201 = case shown="假" w426 {
              tunnel: ["Strength (mT)" 0.0] -> w425
              frame False {
              }
              frame True {
              }
            }
            n202 = Build Array(7.0, w425, "Frequency (Hz)", "Ratio (A/C)", "Direction Angle (deg)", "Pitch Angle (rotating around Origin, deg)", "Pitch Angle (rotating around Constant, deg)") -> (w431:dbl[])
            n203 = shared-variable-write(w436, w434, w431, 1000 ("timeout ms (-1)")) -> (w435:refnum<k21>, w433:errorcluster)  [unwired: 1 out]
          }
          frame "Elliptical Field" {
            n204 = case shown="假" w441 {
              tunnel: ["Ar 2" 0.0] -> w442
              frame False {
              }
              frame True {
              }
            }
            n205 = Build Array(8.0, w442, "wr  2", "pr  2", "dr  2", "ratio", "p_x") -> (w443:dbl[])
            n206 = shared-variable-write(w451, w450, w443, 1000 ("timeout ms (-1)")) -> (w449:refnum<k21>, w448:errorcluster)  [unwired: 1 out]
          }
        }
        "Array" <- w316
        "场强" <- w252
        "dr" <- w250
        n207 = Build Array (concatenate)(w249, w250) -> (w246:ext[])
        "direction angle" <- w246
        n208 = Build Array (concatenate)(w183, w184) -> (w182:ext[])
        n209 = Build Array (concatenate)(w251, w252) -> (w247:dbl[])
        "strength" <- w247
        n210 = Or(x=w317, y="Stop") -> (x .or. y?=w313:bool)
        n211 = Build Array(w248, w247, w246, w245, w240, w244, w243, w242, w236, w232, w213, w212, w199, w195, w190, w182) -> (→"all parameters":ext[][])
        "Numeric 5" <- w53
        "T" <- w53
        "T" <- w53
        "prev_end_point_x" <- w228
        "prev_end_point_y" <- w224
        "prev time" <- w207
      }
    }
    frame #3 {
      # "4. The error -314220 indicates that the other endpoint has been destroyed. The VI ignores this error."
      # "3. Destroy the stream endpoint when you click Stop or when an error occurs."
      # "Close"
      n212 = Flush Stream(8:w461, 11:w464) -> (0:w462:errorcluster, 3:w463:refnum<k21>)  [unwired: 2 in, 1 out]
      n213 = Destroy Stream Endpoint(8:w462, 11:w463) -> (0:w456:errorcluster)
      n214 = Unbundle By Name(w456) -> ("code"=w460:i32)
      n215 = xnode "Error Ring"() -> ("错误输出"=w457:errorcluster)
      n216 = Not Equal?(x=w460, y=-314220) -> (x != y?=w458:bool)
      n217 = Select(t=w456, s=w458, f=w457) -> (s? t:f=→"error out":errorcluster)
    }
  }
